vi "PeriodicTrigger_Main.vi"() -> ()   [LabVIEW 2020]
uses:
  ByValue1_class/ByValue1.lvclass
  PeriodicTrigger/PeriodicTrigger.lvlib
  ByRef1_class/ByRef1.lvclass
  PeriodicTrigger/Triggerable_interface/Triggerable.lvclass
  C:/Projects/InterfacePresentation/PeriodicTrigger/PeriodicTrigger/Triggerable_interface/Triggerable.lvclass
panel:
  out "Measurements":dbl(graph)
  out "By Value Class Triggers":u8(slide) scale=0.0..100.0
  out "Numeric":i32
  out "Triggered":bool
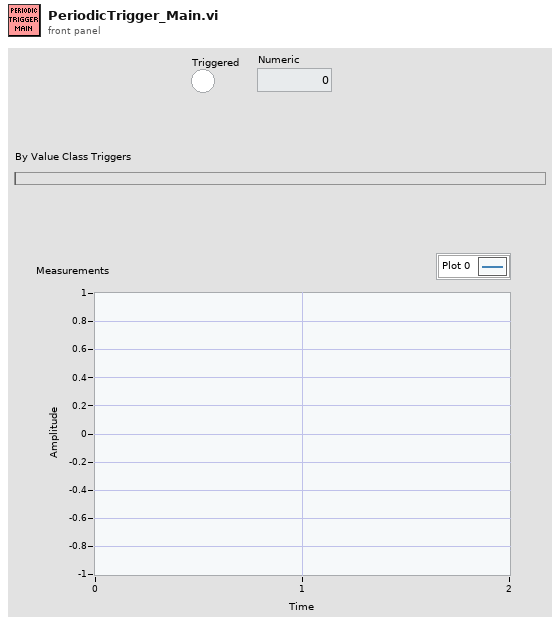
[diagram p1: front panel]
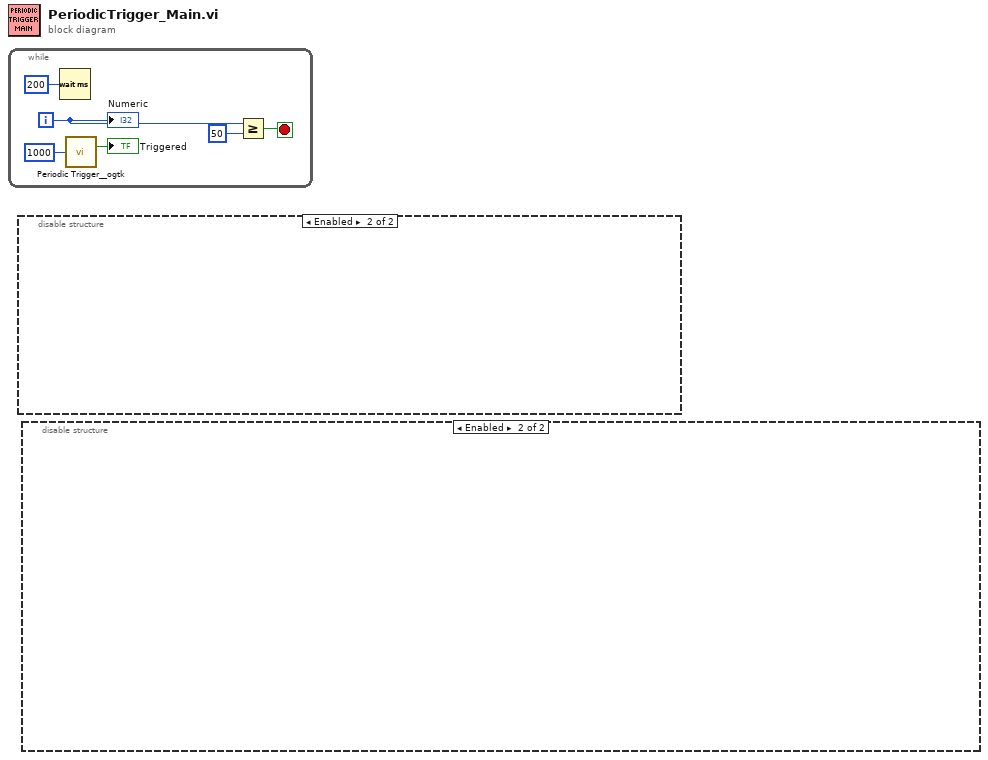
[diagram p0: block diagram]
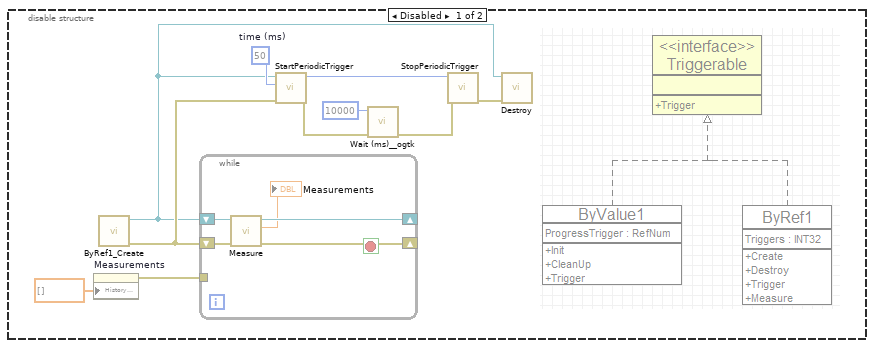
[diagram p2: hidden frame]
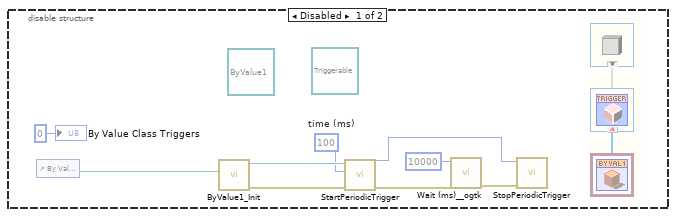
[diagram p3: hidden frame]
diagram:
  n1 = while {
    i -> [w3]
    stop <- w1 stop-if-true
    n2 = Wait (ms)(milliseconds to wait=u32 200) -> ()  [unwired: 1 out]
    n3 = call <userlib>:"Periodic Trigger__ogtk.vi"("time (ms)"=u32 1000) -> ("Triggered"=→"Triggered":bool)  [unwired: 12 in, 2 out]
    n4 = Greater Or Equal?(x=w3, y=50) -> (x >= y?=w1:bool)
    "Numeric" <- w3
  }
  n5 = disable-structure shown="Enabled" {
    frame Disabled {
      (unwired) refnum<class "Triggerable.lvclass"> refnum ("PeriodicTrigger.lvlib:Triggerable")
      (unwired) refnum<class "ByValue1.lvclass"> refnum ("object in")
      w13 = 100  # time (ms)
      n6 = control-ref of="By Value Class Triggers"() -> (w15:refnum<vi>)
      n7 = call "ByValue1_Init.vi"("ProgressTrigger"=w15) -> ("error out"=w12:errorcluster, "object out"=w14:refnum<class "ByValue1.lvclass">)  [unwired: 9 in]
      n8 = call "StartPeriodicTrigger.vi"("error in (no error)"=w12, "time (ms)"=w13, "Triggerable"=w14) -> ("error out"=w11:errorcluster, "TriggerID"=w9:u32)  [unwired: 7 in]
      n9 = call <userlib>:"Wait (ms)__ogtk.vi"("error in (no error)"=w11, "milliseconds to wait"=u32 10000) -> ("error out"=w8:errorcluster)  [unwired: 8 in, 1 out]
      n10 = call "StopPeriodicTrigger.vi"("error in (no error)"=w8, "TriggerID"=w9) -> ()  [unwired: 9 in, 1 out]
      "By Value Class Triggers" <- u8 0 ("By Value Class Triggers")
    }
    frame Enabled {
    }
  }
  n11 = disable-structure shown="Enabled" {
    frame Disabled {
      w25 = 50  # time (ms)
      n12 = property on="Measurements" class="WFChart (strict)"("History Data"=dbl[] []) -> (error out=w21:errorcluster)  [unwired: 2 in, 1 out]
      n13 = call "ByRef1_Create.vi"() -> ("error out"=w24:errorcluster, "reference out"=w19:refnum<class "ByRef1.lvclass">)  [unwired: 10 in]
      n14 = while {
        shift-right: [w29] -> _
        shift-left: w19 -> [w30]
        shift-right: [w27] -> _
        shift-left: w24 -> [w28]
        tunnel: w21 -> [_]
        stop <- w27 stop-if-true
        n15 = call-dynamic "Measure.vi"("Error In"=w28, "reference in"=w30) -> ("Error Out"=w27:errorcluster, "Measurement"=→"Measurements":dbl, "reference out"=w29:refnum<class "ByRef1.lvclass">)  [unwired: 7 in]
      }
      n16 = call "StartPeriodicTrigger.vi"("error in (no error)"=w24, "time (ms)"=w25, "Triggerable"=w19) -> ("error out"=w17:errorcluster, "TriggerID"=w23:u32)  [unwired: 7 in]
      n17 = call <userlib>:"Wait (ms)__ogtk.vi"("error in (no error)"=w17, "milliseconds to wait"=u32 10000) -> ("error out"=w16:errorcluster)  [unwired: 8 in, 1 out]
      n18 = call "StopPeriodicTrigger.vi"("error in (no error)"=w16, "TriggerID"=w23) -> ("error out"=w20:errorcluster)  [unwired: 9 in]
      n19 = call-dynamic "Destroy.vi"("error in (no error)"=w20, "reference in"=w19) -> ()  [unwired: 8 in, 2 out]
    }
    frame Enabled {
    }
  }
